vi "wrap data.vi"(10 "identifier":string, 11 "data to wrap":string) -> (3 "wrapped data":string)   [LabVIEW 2013, in "NISE_CEF_serializable configuration.lvclass"]
doc: "Generates a packed dataset of the form:\n<identifier>data to wrap</identifier>"
uses:
  NISE_CEF_serializable configuration.lvclass
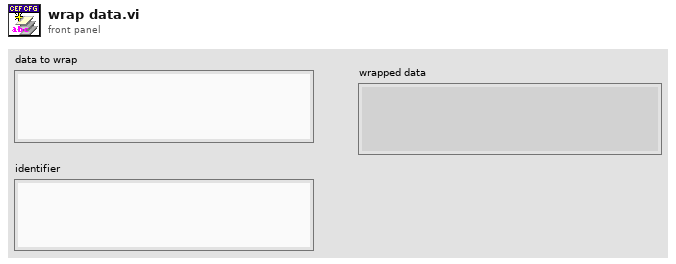
[diagram p1: front panel]
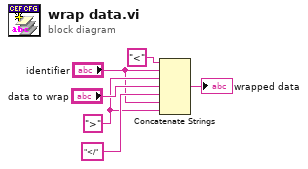
[diagram p0: block diagram]
diagram:
  w2 = ">" ("string")
  n1 = Concatenate Strings("<" ("string"), "identifier", w2, "data to wrap", "</" ("string"), "identifier", w2) -> (→"wrapped data":string)
